vi "reponsegetport.vi"(8 "error in (no error)":errorcluster, 11 "Arduino in":refnum<class "Arduino.lvclass">) -> (0 "error out":errorcluster, 2 "String":string, 3 "Arduino out":refnum<class "Arduino.lvclass">)   [LabVIEW 2019, in "Arduino.lvclass"]
uses:
  Arduino.lvclass
  Arduino.lvclass/Arduino.ctl
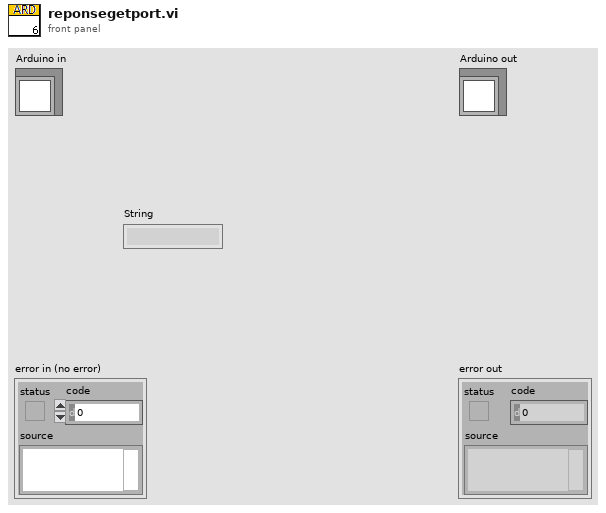
[diagram p1: front panel]
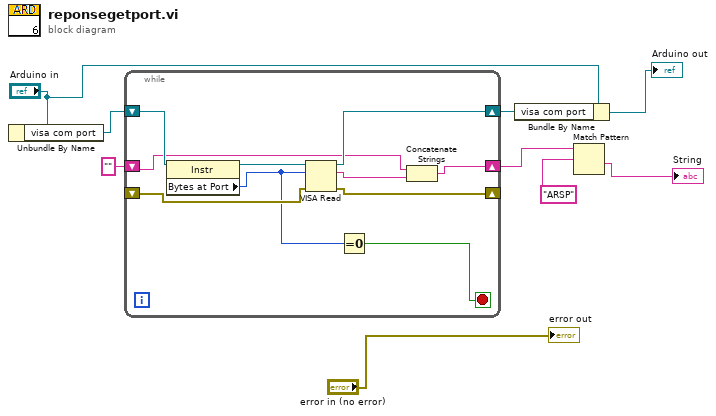
[diagram p0: block diagram]
diagram:
  n1 = Unbundle By Name("Arduino in") -> ("visa com port"=w7:refnum<visa-resource-name>)
  n2 = while {
    shift-right: [w17] -> w6
    shift-left: w7 -> [w19]
    shift-right: [w16] -> _
    shift-left: _ -> [w15]
    shift-right: [w13] -> w4
    shift-left: "" -> [w12]
    stop <- w10 stop-if-true
    n3 = property class="Instr"(reference=w19) -> (reference out=w18:refnum<visa-resource-name>, "Bytes at Port"=w11:u32)  [unwired: 1 in, 1 out]
    n4 = VISA Read(VISA resource name=w18, byte count=w11, error in (no error)=w15) -> (VISA resource name out=w17:refnum<visa-resource-name>, read buffer=w14:string, error out=w16:errorcluster)  [unwired: 1 out]
    n5 = Equal To 0?(x=w11) -> (x = 0?=w10:bool)
    n6 = Concatenate Strings(w12, w14) -> (w13:string)
  }
  n7 = Bundle By Name(cluster="Arduino in", "visa com port"=w6) -> (→"Arduino out":refnum<class "Arduino.lvclass">)
  n8 = Match Pattern(string=w4, regular expression="ARSP") -> (after substring=→"String":string)  [unwired: 1 in, 3 out]
  "error out" <- "error in (no error)"
